vi "rs3 get frame profile.vi"(8 "error in (no error)":errorcluster, 11 "Frame":u64) -> (0 "error out":errorcluster, 1 "stream profile":u64, 2 "error out":u64, 3 "frame out":u64)   [LabVIEW 2018, in "libRealSense3.lvlib"]
doc: "Returns the stream profile pointer for the captured FRAME. \nUse the profile handle to get more info about the captured frame, using Get_Profile_data"
uses:
  libRealSense3.lvlib
  realsense2.dll
panel:
  # "RS3 Get Frame Profile"
  # "(C) Intel Corp., 2017  AGJ"
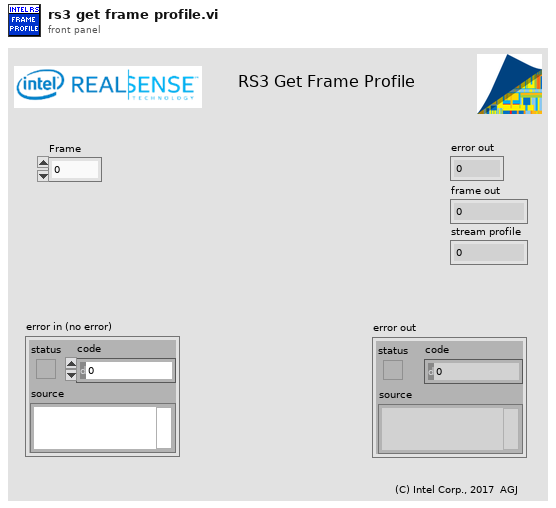
[diagram p1: front panel]
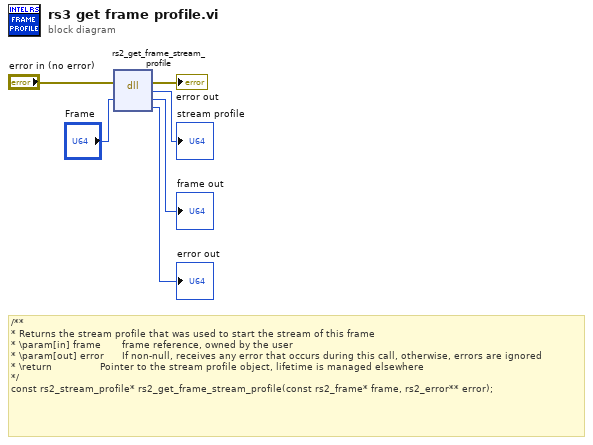
[diagram p0: block diagram]
diagram:
  # "/**\n* Returns the stream profile that was used to start the stream of this frame\n* \\param[in] frame       frame reference, owned by the user\n* \\param[out] error      If non-null, receives any error that occurs during this call, otherwise, errors are ignored\n* \\return                Pointer to the stream profile object, lifetime is managed elsewhere\n*/\nconst rs2_stream_profile* rs2_get_frame_stream_profile(const rs2_frame* frame, rs2_error** error);"
  n1 = dll-call lib="C:/Users/aaron.jencks/Documents/GitHub/emerson_seed_object_detection/LabVIEW/Projects/Paul's Video Viewer/Classes/Realsense Cam/realsense_wrapper_api/realsense2.dll" fn="rs2_get_frame_stream_profile"(error in="error in (no error)", "frame"="Frame") -> (error out=→"error out":errorcluster, "stream profile"=→"stream profile":u64, "frame"=→"frame out":u64, "error"=→"error out":u64)  [unwired: 3 in, 1 out]
